vi "clog2.vi"() -> ()   [LabVIEW 2015]
panel:
  out "ceil(x): smallest int >= x":dbl
  out "clog2":i32
  in  "Input":u32
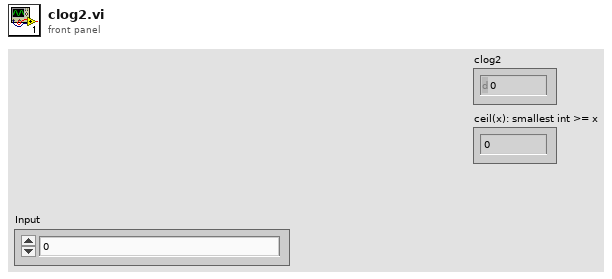
[diagram p1: front panel]
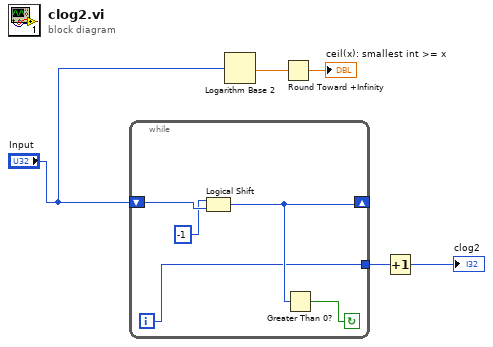
[diagram p0: block diagram]
diagram:
  n1 = while {
    shift-right: [w8] -> _
    shift-left: "Input" -> [w10]
    tunnel: [w6] -> w5
    i -> [w6]
    stop <- w7 continue-if-true
    n2 = Logical Shift(y=i16 -1, x=w10) -> (x << y=w8:u32)
    n3 = Greater Than 0?(x=w8) -> (x > 0?=w7:bool)
  }
  n4 = Logarithm Base 2(1:"Input") -> (0:w3:dbl)
  n5 = Round Toward +Infinity(x=w3) -> (ceil(x): smallest int >= x=→"ceil(x): smallest int >= x":dbl)
  n6 = Increment(x=w5) -> (x+1=→"clog2":i32)
